vi "UTM To Image.vi"(3 "error in":errorcluster, 4 "Image Descriptor":T2={"Upper-Left Corner Coordinates"={"UTM Zone"=0.0, "Hemisphere"=enum."North", "East"=0.0, "North"=0.0}, "Meters/Pixel"=42.294203}, 5 "UTM Location":T1) -> (0 "error out":errorcluster, 1 "Y":i32, 2 "X":i32)   [LabVIEW 2011]
uses:
  0-Image Descriptor.ctl
  2-Think/2 Typedefs/UTM Location.ctl
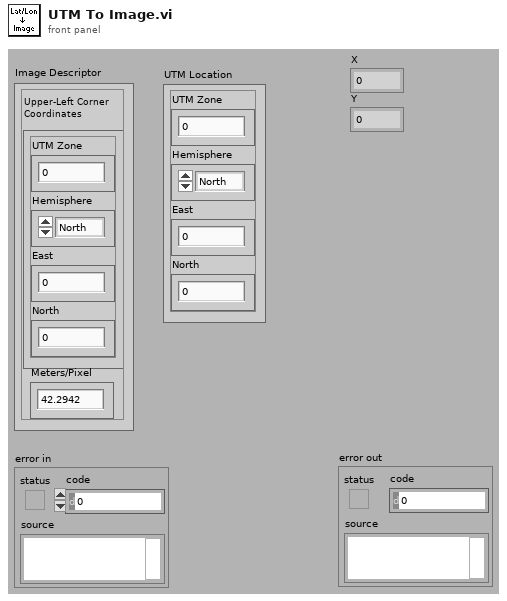
[diagram p1: front panel]
types:
  T1 = typedef "UTM Location.ctl" = cluster{"UTM Zone":dbl, "Hemisphere":enum16{"North", "South"}, "East":dbl, "North":dbl}
  T2 = typedef "0-Image Descriptor.ctl" = cluster{"Upper-Left Corner Coordinates":T1, "Meters/Pixel":dbl}
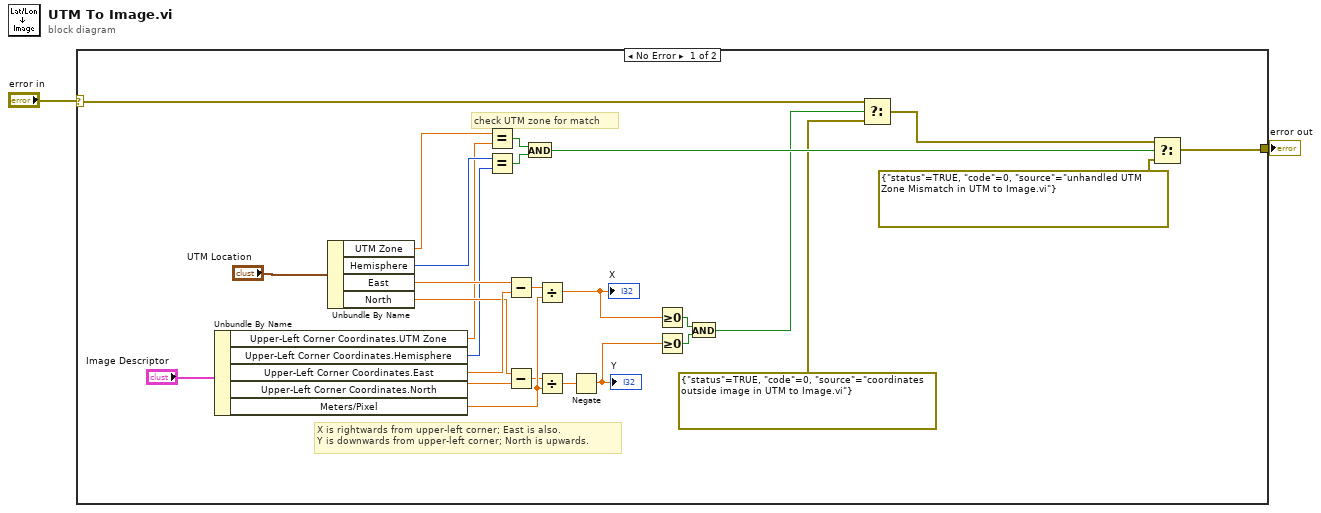
[diagram p0: block diagram]
diagram:
  n1 = case shown="No Error" "error in" {
    selector: "error in" -> [w4 w30]
    tunnel: [w11 w30] -> w1
    frame No Error {
      # "check UTM zone for match"
      # "X is rightwards from upper-left corner; East is also.\nY is downwards from upper-left corner; North is upwards."
      n2 = Unbundle By Name("Image Descriptor") -> ("Upper-Left Corner Coordinates.UTM Zone"=w17:dbl, "Upper-Left Corner Coordinates.Hemisphere"=w18:enum16{"North", "South"}, "Upper-Left Corner Coordinates.East"=w27:dbl, "Upper-Left Corner Coordinates.North"=w26:dbl, "Meters/Pixel"=w25:dbl)
      n3 = Unbundle By Name("UTM Location") -> ("UTM Zone"=w16:dbl, "Hemisphere"=w19:enum16{"North", "South"}, "East"=w22:dbl, "North"=w21:dbl)
      n4 = Equal?(x=w16, y=w17) -> (x = y?=w15:bool)
      n5 = Equal?(x=w19, y=w18) -> (x = y?=w14:bool)
      n6 = Subtract(x=w22, y=w27) -> (x-y=w20:dbl)
      n7 = Subtract(x=w21, y=w26) -> (x-y=w24:dbl)
      n8 = And(x=w15, y=w14) -> (x .and. y?=w13:bool)
      n9 = Divide(x=w20, y=w25) -> (x/y=w10:dbl)
      "X" <- w10
      n10 = Divide(x=w24, y=w25) -> (x/y=w29:dbl)
      n11 = Negate(x=w29) -> (-x=w9:dbl)
      "Y" <- w9
      n12 = Greater Or Equal To 0?(x=w10) -> (x >= 0?=w7:bool)
      n13 = Greater Or Equal To 0?(x=w9) -> (x >= 0?=w8:bool)
      n14 = And(x=w7, y=w8) -> (x .and. y?=w6:bool)
      n15 = Select(t=w4, s=w6, f=errorcluster {"status"=TRUE, "code"=0, "source"="coordinates outside image in UTM to Image.vi"} ("error IO")) -> (s? t:f=w3:errorcluster)
      n16 = Select(t=w3, s=w13, f=errorcluster {"status"=TRUE, "code"=0, "source"="unhandled UTM Zone Mismatch in UTM to Image.vi"} ("error IO")) -> (s? t:f=w11:errorcluster)
    }
    frame Error {
    }
  }
  "error out" <- w1
